vi "AD（光斑）40M.vi"(8 "N-length":dbl, 9 "M-length":dbl, 10 "hDevice":i32, 11 "pulDDR2Length":u32) -> (0 "幅频谱":dbl[](graph), 1 "时域谱":dbl[](graph), 3 "hDevice out":i32)   [LabVIEW 2016]
uses:
  <vilib>/Analysis/2dsp.llb/Real FFT.vi
  INF/amd64/PCI8502_32.dll
  <vilib>/Analysis/NI_AALPro.lvlib
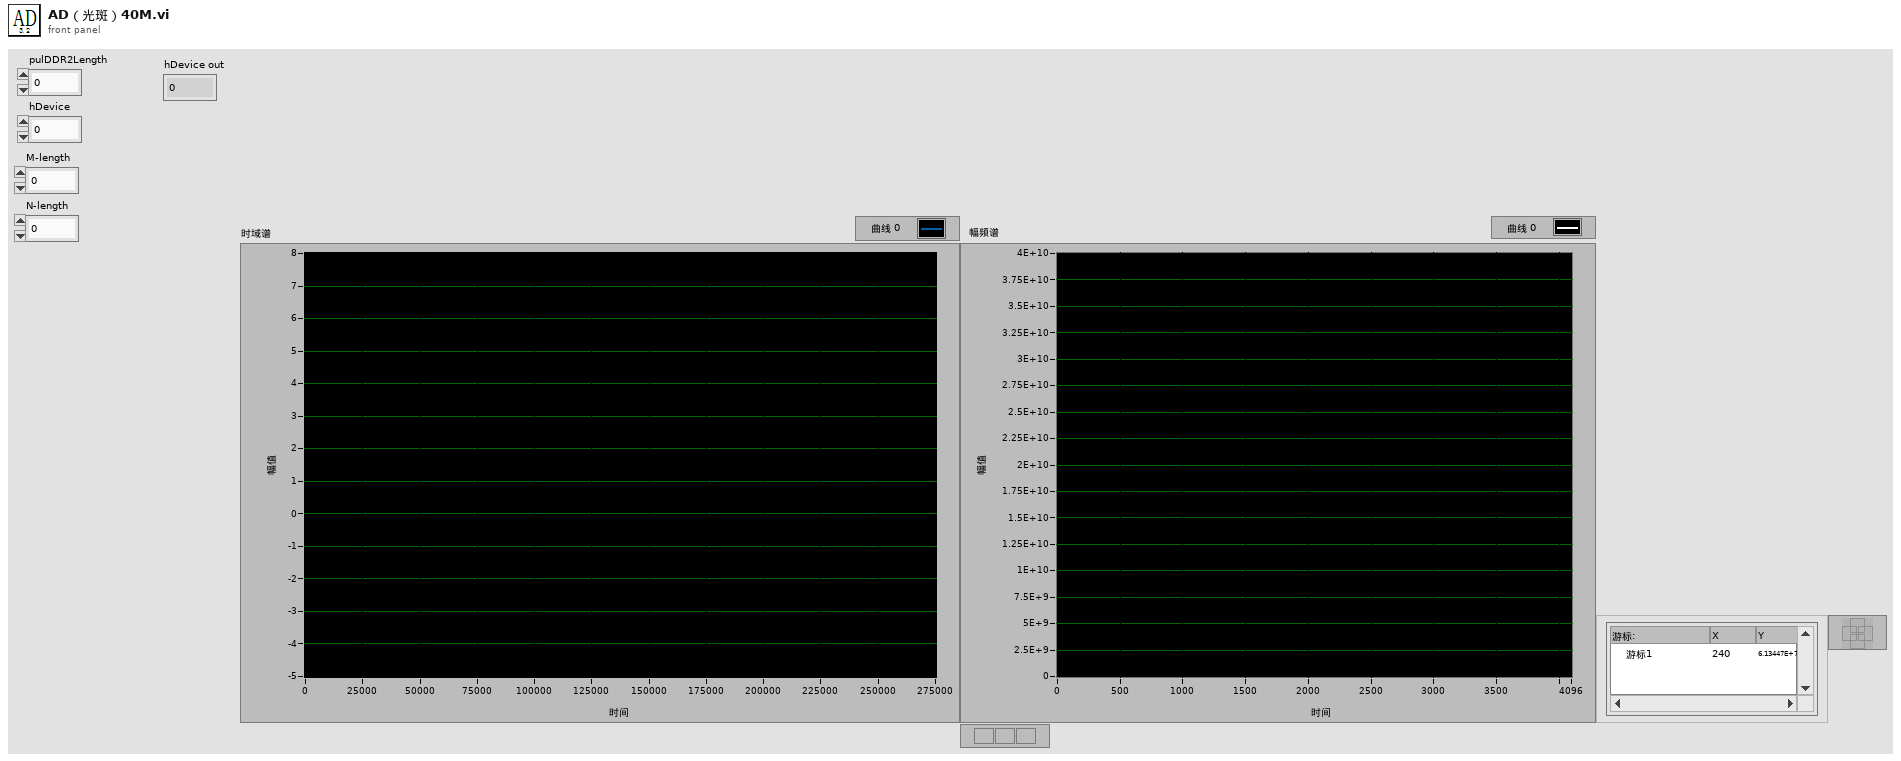
[diagram p1: front panel]
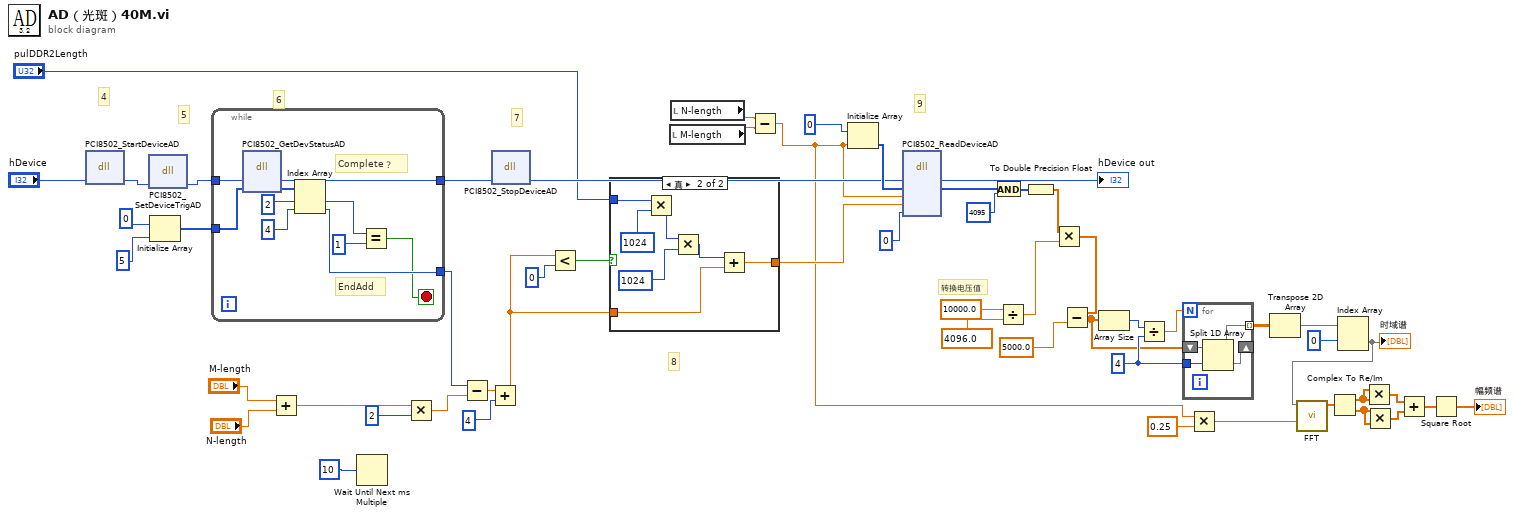
[diagram p0: block diagram]
diagram:
  w23 = 4
  # "9"
  # "8"
  # "7"
  # "6"
  # "5"
  # "4"
  # "转换电压值"
  n1 = dll-call lib="PTH2]abs CUsersH301Desktopart闭环扫描程序采集卡控制INFamd64\nPCI8502_32" fn="PCI8502_StartDeviceAD" label="StartDeviceAD"("hDevice"="hDevice") -> ("hDevice"=w54:i32)  [unwired: 4 in, 2 out]
  n2 = dll-call lib="PTH2]abs CUsersH301Desktopart闭环扫描程序采集卡控制INFamd64\nPCI8502_32" fn="PCI8502_SetDeviceTrigAD" label="SetDeviceTrigAD"("hDevice"=w54) -> ("hDevice"=w31:i32)  [unwired: 4 in, 2 out]
  n3 = Initialize Array(0, 5) -> (w28:i32[])
  n4 = while {
    tunnel: [w60] -> w27
    tunnel: w31 -> [w59]
    tunnel: w28 -> [w58]
    tunnel: [w57] -> w25
    stop <- w56 stop-if-true
    # "EndAdd"
    # "Complete？"
    n5 = dll-call lib="PTH2aabs CUsersH301Desktopart闭环扫描程序采集卡控制INFamd64PCI8502_32.dll" fn="PCI8502_GetDevStatusAD" label="GetDevStatusAD"("hDevice"=w59, "pADStatus"=w58) -> ("hDevice"=w57:i32, "pADStatus"=w62:i32[])  [unwired: 4 in, 2 out]
    n6 = Index Array(array=w62, index #1=2, index #2=4) -> (element #1=w64:i32, element #2=w60:i32)
    n7 = Equal?(x=w64, y=1) -> (x = y?=w56:bool)
  }
  n8 = Add(x="M-length", y="N-length") -> (x+y=w26:dbl)
  n9 = Wait Until Next ms Multiple(millisecond multiple=u32 10) -> ()  [unwired: 1 out]
  n10 = Multiply(x=w26, y=u32 2) -> (x*y=w39:dbl)
  n11 = Subtract(x=w27, y=w39) -> (x-y=w41:dbl)
  n12 = Add(x=w41, y=u32 4) -> (x+y=w36:dbl)
  n13 = dll-call lib="PTH2]abs CUsersH301Desktopart闭环扫描程序采集卡控制INFamd64\nPCI8502_32" fn="PCI8502_StopDeviceAD" label="StopDeviceAD"("hDevice"=w25) -> ("hDevice"=w42:i32)  [unwired: 4 in, 2 out]
  n14 = Less?(x=w36, y=u32 0) -> (x < y?=w32:bool)
  n15 = case shown="真" w32 {
    tunnel: w36 -> [w66 w69]
    tunnel: [w66 w68] -> w37
    tunnel: "pulDDR2Length" -> [_ w67]
    frame False {
    }
    frame True {
      n16 = Multiply(x=w67, y=u32 1024) -> (x*y=w72:u32)
      n17 = Multiply(x=w72, y=u32 1024) -> (x*y=w70:u32)
      n18 = Add(x=w70, y=w69) -> (x+y=w68:dbl)
    }
  }
  n19 = local read "M-length"() -> (w13:dbl)
  n20 = local read "N-length"() -> (w14:dbl)
  n21 = Subtract(x=w14, y=w13) -> (x-y=w11:dbl)
  n22 = Initialize Array(0, w11) -> (w43:i32[])
  n23 = dll-call lib="PTH2]abs CUsersH301Desktopart闭环扫描程序采集卡控制INFamd64\nPCI8502_32" fn="PCI8502_ReadDeviceAD" label="ReadDeviceAD"("hDevice"=w42, "ADBuffer"=w43, "nReadSizeWords"=w11, "ulStartAddr"=w37, "nRetSizeWords"=0) -> ("hDevice"=→"hDevice out":i32, "ADBuffer"=w34:u16[])  [unwired: 7 in, 2 out]
  n24 = And(x=w34, y=4095) -> (x .and. y?=w45:i32[])
  n25 = Divide(x=10000.0, y=4096.0) -> (x/y=w47:dbl)
  n26 = To Double Precision Float(number=w45) -> (double precision float=w48:dbl[])
  n27 = Multiply(x=w48, y=w47) -> (x*y=w46:dbl[])
  n28 = Subtract(x=w46, y=5000.0) -> (x-y=w21:dbl[])
  n29 = Array Size(array=w21) -> (size(s)=w24:i32)
  n30 = Divide(x=w24, y=w23) -> (x/y=w22:dbl)
  n31 = for {
    N: w22 -> [_]
    tunnel: w23 -> [w77]
    shift-right: [w75] -> _
    shift-left: w21 -> [w76]
    tunnel: [w74] -> w20 mode=indexing
    n32 = Split 1D Array(array=w76, index=w77) -> (first subarray=w74:dbl[], second subarray=w75:dbl[])
  }
  n33 = Multiply(x=w11, y=0.25) -> (x*y=w9:dbl)
  n34 = Transpose 2D Array(2D array=w20) -> (transposed array=w10:dbl[][])
  n35 = Index Array(array=w10, index (row)=0 ("索引 (行)")) -> (element=w19:dbl[])  [unwired: 1 in]
  "时域谱" <- w19
  n36 = call-poly <vilib>:"FFT.vi"("FFT size"=w9, "X"=w19) -> ("FFT {X}"=w8:cdb[])  [unwired: 8 in, 1 out]
  n37 = Complex To Re/Im(x + iy=w8) -> (x=w7:dbl[], y=w6:dbl[])
  n38 = Multiply(x=w7, y=w7) -> (x*y=w5:dbl[])
  n39 = Multiply(x=w6, y=w6) -> (x*y=w4:dbl[])
  n40 = Add(x=w5, y=w4) -> (x+y=w3:dbl[])
  n41 = Square Root(x=w3) -> (sqrt(x)=→"幅频谱":dbl[])
